vi "RF_SetIQCaptureBuffer.vi"(7 "RFIndex":u32, 8 "error in (no error)":errorcluster) -> (0 "error out":errorcluster, 3 "return":i32, 10 "Q":i16[](array[numeric]), 11 "I":i16[](array[numeric]))   [LabVIEW 2018]
uses:
  Common/Driver/rd.dll
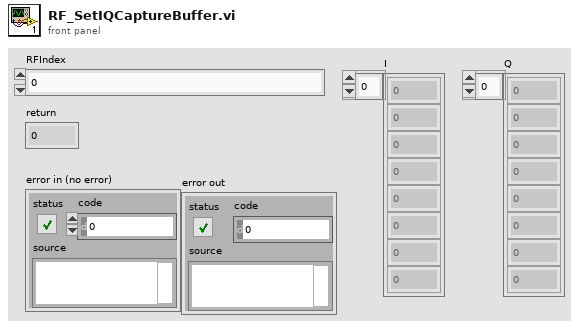
[diagram p1: front panel]
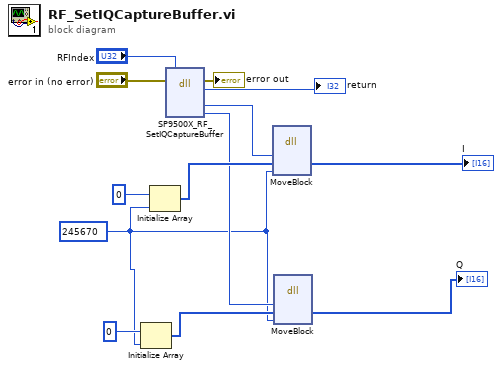
[diagram p0: block diagram]
diagram:
  w2 = 245670 ("size")
  n1 = Initialize Array(0, w2) -> (w3:i32[])
  n2 = Initialize Array(0, w2) -> (w7:i32[])
  n3 = dll-call lib="C:/rd/LabVIEW/Common/Driver/rd.dll" fn="SP9500X_RF_SetIQCaptureBuffer"(error in="error in (no error)", "RFIndex"="RFIndex") -> (error out=→"error out":errorcluster, "return"=→"return":i32, "I"=w9:i16, "Q"=w5:i16)  [unwired: 5 in, 1 out]
  n4 = dll-call lib="LabVIEW" fn="MoveBlock"("address"=w9, "I"=w7, "size"=w2) -> ("I"=→"I":i32[])  [unwired: 6 in, 2 out]
  n5 = dll-call lib="LabVIEW" fn="MoveBlock"("address"=w5, "Q"=w3, "size"=w2) -> ("Q"=→"Q":i32[])  [unwired: 6 in, 2 out]
